vi "Write Digital.vi"   [LabVIEW 2014, in "SLSC configuration Shared.lvlib"]
doc: "Writes the value of the pins on the chip."
uses:
  SLSC configuration Shared.lvlib
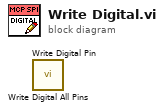
[diagram p0: block diagram]
diagram:
  n1 = call "Write Digital All Pins.vi"() -> ()  [unwired: 9 in, 3 out]
  n2 = call "Write Digital Pin.vi"() -> ()  [unwired: 9 in, 3 out]
